vi "CTL_SpecCheckRev3.vi"(6 "Max Index":i32=12, 7 "Drain!Fill":bool, 8 "Level IN inches":dbl=5.0, 9 "Index":i32=3, 10 "ChA/!ChB":bool, 11 "Full Cfg":T3) -> (0 "Measure":dbl, 1 "Set Point":dbl, 3 "In Range?":bool=TRUE)   [LabVIEW 2024]
uses:
  Control Definitions/Ded LUT_Status.ctl
  Control Definitions/Def Spec RNG.ctl
  Control Definitions/Def Bench Status.ctl
  Control Definitions/Def PumpCtlRefs.ctl
  Control Definitions/Def BenchCfg.ctl
  Control Definitions/Def FullCfg.ctl
  Control Definitions/Def_PumpSpeed.ctl
panel:
  out "Spec Range Out":T1
  out "error out":errorcluster
  in  "error in (no error)":errorcluster
  # "In Range = TRUE when"
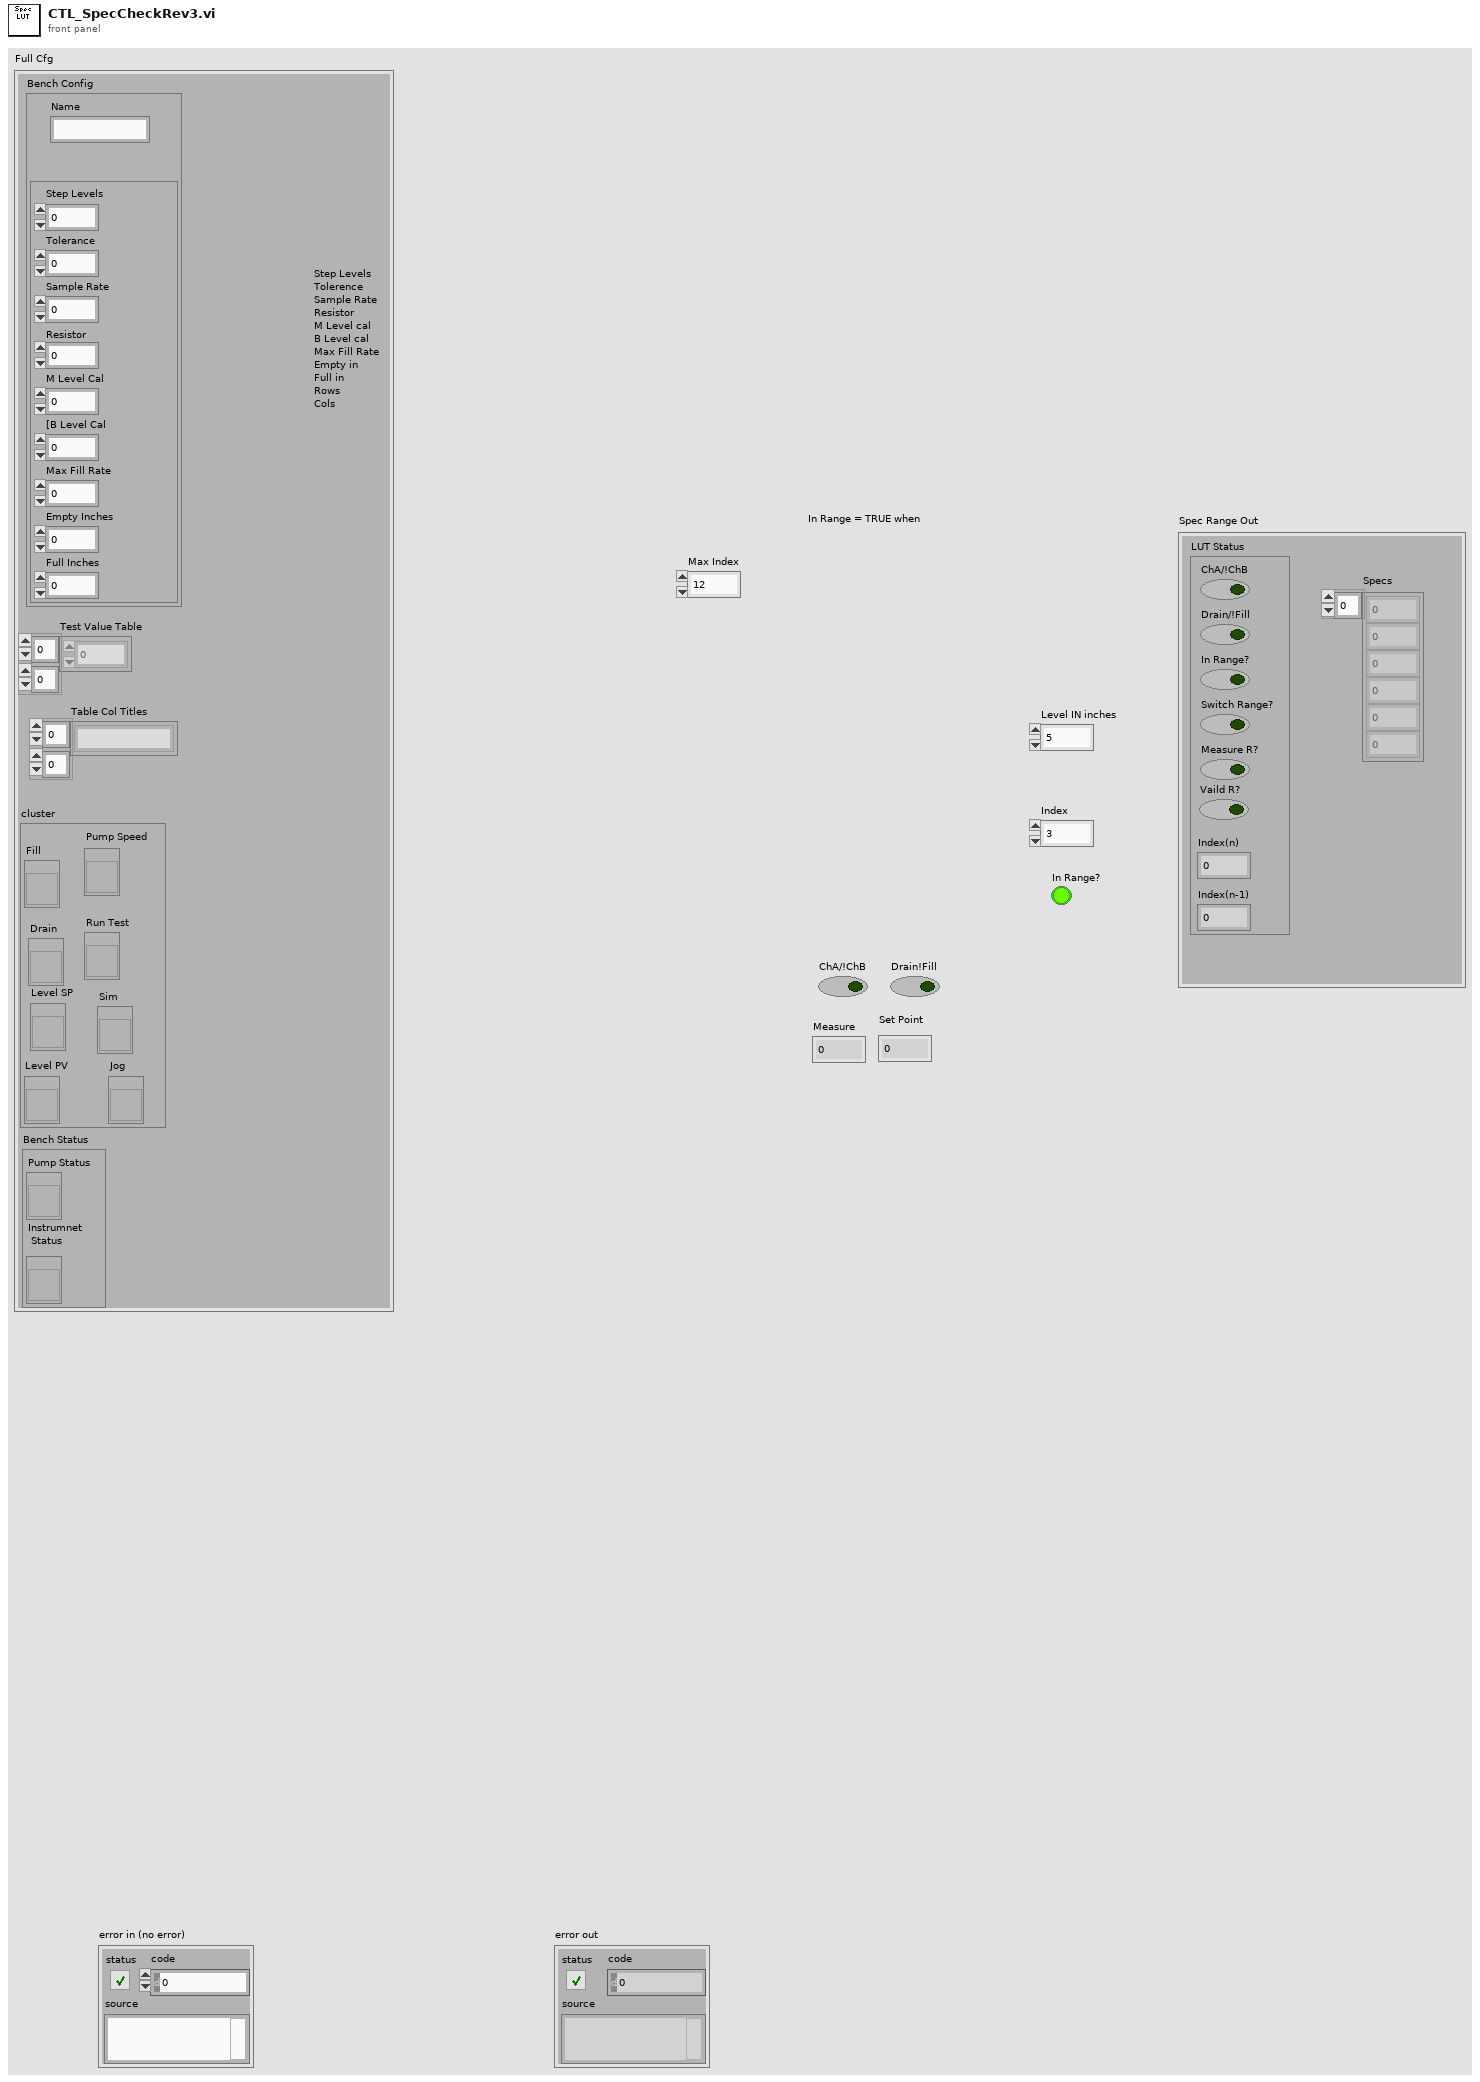
[diagram p1: front panel]
types:
  T1 = typedef "Def Spec RNG.ctl" = cluster{"Specs":dbl[], "LUT Status":T2}
  T2 = typedef "Ded LUT_Status.ctl" = cluster{"ChA/!ChB":bool, "Drain/!Fill":bool, "In Range?":bool, "Switch Range?":bool, "Measure R?":bool, "Vaild R?":bool, "Index(n)":i32, "Index(n-1)":i32}
  T3 = typedef "Def FullCfg.ctl" = cluster{"Bench Config":T4, "Test Value Table ":dbl[][], "Table Col Titles":string[][], "cluster":T5, "Bench Status":T6}
  T4 = typedef "Def BenchCfg.ctl" = cluster{"Name":string, cluster{"Step Levels":dbl, "Tolerance":dbl, "Sample Rate":dbl, "Resistor":dbl, "M Level Cal":dbl, "[B Level Cal":dbl, "Max Fill Rate":dbl, "Empty Inches":dbl, "Full Inches":dbl}}
  T5 = typedef "Def PumpCtlRefs.ctl" = cluster{"Fill ":refnum<vi>, "Drain":refnum<vi>, "Level PV":refnum<vi>, "Pump Speed":refnum<vi>, "Run Test":refnum<vi>, "Sim":refnum<vi>, "Jog":refnum<vi>, "Level SP":refnum<vi>}
  T6 = typedef "Def Bench Status.ctl" = cluster{"Pump Status":refnum<vi>, "Instrumnet\n Status":refnum<vi>}
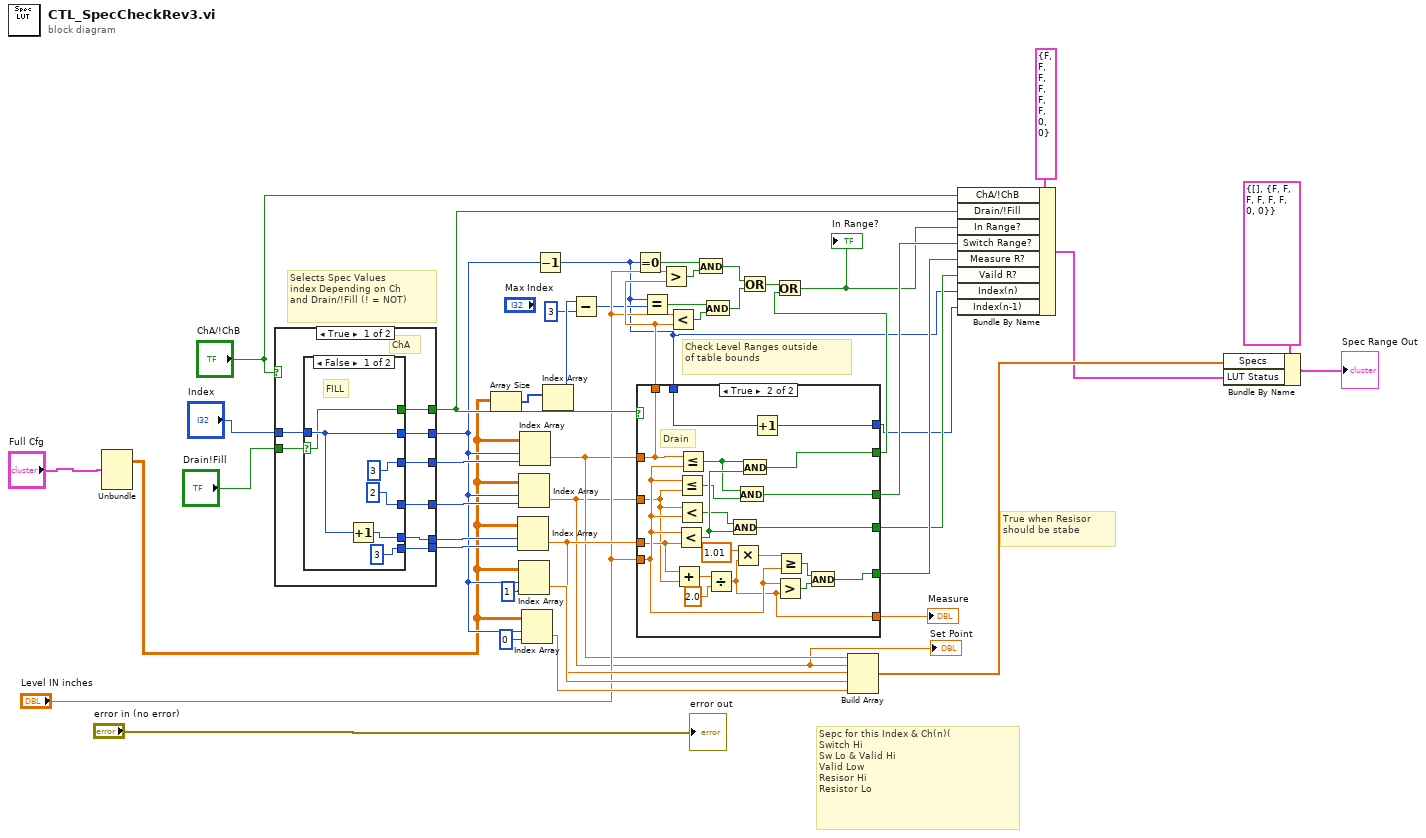
[diagram p0: block diagram]
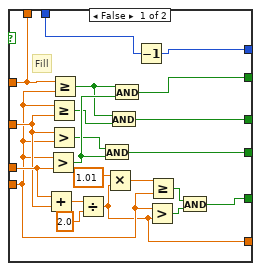
[diagram p2: hidden frame]
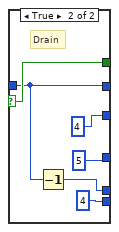
[diagram p3: hidden frame]
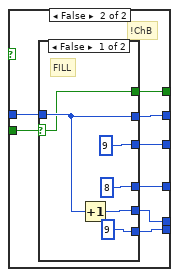
[diagram p4: hidden frame]
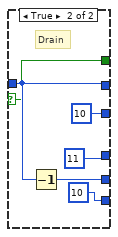
[diagram p5: hidden frame]
diagram:
  # "Selects Spec Values\nindex Depending on Ch\nand Drain/!Fill (! = NOT)"
  # "True when Resisor \nshould be stabe"
  # "Sepc for this Index & Ch(n)(\nSwitch Hi\nSw Lo & Valid Hi  \nValid Low\nResisor Hi\nResistor Lo"
  # "Check Level Ranges outside \nof table bounds"
  n1 = Unbundle("Full Cfg") -> ("Test Value Table"=w15:dbl[][])  [unwired: 4 out]
  n2 = case shown="True" "ChA/!ChB" {
    tunnel: "Drain!Fill" -> [w53 w67]
    tunnel: "Index" -> [w52 w73]
    tunnel: [w51 w72] -> w21
    tunnel: [w50 w71] -> w42
    tunnel: [w49 w70] -> w41
    tunnel: [w48 w69] -> w40
    tunnel: [w47 w68] -> w23
    tunnel: [w46 w66] -> w27
    frame True {
      # "ChA"
      n3 = case shown="False" w53 {
        selector: w53 -> [w54 w62]
        tunnel: [3 ("disabled index (col)") 4 ("disabled index (col)")] -> w47
        tunnel: [3 ("disabled index (col)") 4 ("disabled index (col)")] -> w49
        tunnel: w52 -> [w55 w60]
        tunnel: [w55 w60] -> w51
        tunnel: [w57 w61] -> w50
        tunnel: [2 ("disabled index (col)") 5 ("disabled index (col)")] -> w48
        tunnel: [w54 w62] -> w46
        frame False {
          # "FILL"
          n4 = Increment(x=w55) -> (x+1=w57:i32)
        }
        frame True {
          # "Drain"
          n5 = Decrement(x=w60) -> (x-1=w61:i32)
        }
      }
    }
    frame False {
      # "!ChB"
      n6 = case shown="False" w67 {
        selector: w67 -> [w74 w80]
        tunnel: [9 ("disabled index (col)") 10 ("disabled index (col)")] -> w68
        tunnel: [9 ("disabled index (col)") 10 ("disabled index (col)")] -> w70
        tunnel: w73 -> [w75 w81]
        tunnel: [w75 w81] -> w72
        tunnel: [w77 w83] -> w71
        tunnel: [8 ("disabled index (col)") 11 ("disabled index (col)")] -> w69
        tunnel: [w74 w80] -> w66
        frame False {
          # "FILL"
          n7 = Increment(x=w75) -> (x+1=w77:i32)
        }
        frame True {
          # "Drain"
          n8 = Decrement(x=w81) -> (x-1=w83:i32)
        }
      }
    }
  }
  n9 = Array Size(array=w15) -> (size(s)=w19:i32[])
  n10 = Index Array(array=w15, index (row)=w42, index (col)=w23) -> (element=w37:dbl)
  n11 = Index Array(array=w15, index (row)=w21, index (col)=w40) -> (element=w8:dbl)
  "Set Point" <- w8
  n12 = Index Array(array=w15, index (row)=w21, index (col)=1 ("disabled index (col)")) -> (element=w39:dbl)
  n13 = Index Array(array=w15, index (row)=w21, index (col)=w41) -> (element=w9:dbl)
  n14 = Index Array(array=w15, index (row)=w21, index (col)=0 ("disabled index (col)")) -> (element=w38:dbl)
  n15 = Decrement(x=w21) -> (x-1=w6:i32)
  n16 = Index Array(array=w19) -> (element=w18:i32)  [unwired: 1 in]
  n17 = Subtract(x=w18, y=3) -> (x-y=w16:i32)
  n18 = Equal To 0?(x=w6) -> (x = 0?=w33:bool)
  n19 = case shown="True" w27 {
    tunnel: "Level IN inches" -> [w91 w114]
    tunnel: w9 -> [w89 w112]
    tunnel: w37 -> [w99 w111]
    tunnel: [w106 w127] -> w29
    tunnel: w8 -> [w98 w110]
    tunnel: [w103 w124] -> w13
    tunnel: [w100 w121] -> w26
    tunnel: [w90 w113] -> w25
    tunnel: [w89 w112] -> w24
    tunnel: [w88 w109] -> w11
    tunnel: [w87 w108] -> w5
    tunnel: w6 -> [w86 w107]
    frame False {
      # "Fill"
      n20 = Add(x=w99, y=w98) -> (x+y=w97:dbl)
      n21 = Greater?(x=w91, y=w99) -> (0:w105:bool)
      n22 = Greater Or Equal?(x=w91, y=w98) -> (x >= y?=w101:bool)
      n23 = Greater?(x=w98, y=w91) -> (0:w104:bool)
      n24 = Greater Or Equal?(x=w89, y=w91) -> (x >= y?=w102:bool)
      n25 = Divide(x=w97, y=2.0) -> (x/y=w88:dbl)
      n26 = And(x=w104, y=w105) -> (x .and. y?=w103:bool)
      n27 = Multiply(x=1.01, y=w88) -> (x*y=w92:dbl)
      n28 = And(x=w102, y=w101) -> (x .and. y?=w100:bool)
      n29 = And(x=w102, y=w105) -> (x .and. y?=w106:bool)
      n30 = Decrement(x=w86) -> (x-1=w87:i32)
      n31 = Greater?(x=w91, y=w88) -> (0:w95:bool)
      n32 = Greater Or Equal?(x=w92, y=w91) -> (x >= y?=w94:bool)
      n33 = And(x=w94, y=w95) -> (x .and. y?=w90:bool)
    }
    frame True {
      # "Drain"
      n34 = Add(x=w111, y=w110) -> (x+y=w120:dbl)
      n35 = Less?(x=w114, y=w111) -> (x < y?=w126:bool)
      n36 = Less Or Equal?(x=w114, y=w110) -> (x <= y?=w122:bool)
      n37 = Less?(x=w110, y=w114) -> (x < y?=w125:bool)
      n38 = Less Or Equal?(x=w112, y=w114) -> (x <= y?=w123:bool)
      n39 = Divide(x=w120, y=2.0) -> (x/y=w109:dbl)
      n40 = And(x=w125, y=w126) -> (x .and. y?=w124:bool)
      n41 = Multiply(x=1.01, y=w109) -> (x*y=w115:dbl)
      n42 = And(x=w123, y=w122) -> (x .and. y?=w121:bool)
      n43 = And(x=w123, y=w126) -> (x .and. y?=w127:bool)
      n44 = Increment(x=w107) -> (x+1=w108:i32)
      n45 = Greater?(x=w114, y=w109) -> (0:w118:bool)
      n46 = Greater Or Equal?(x=w115, y=w114) -> (x >= y?=w117:bool)
      n47 = And(x=w117, y=w118) -> (x .and. y?=w113:bool)
    }
  }
  "Measure" <- w11
  n48 = Equal?(x=w6, y=w16) -> (x = y?=w35:bool)
  n49 = Greater?(x="Level IN inches", y=w24) -> (0:w34:bool)
  n50 = Less?(x="Level IN inches", y=w24) -> (x < y?=w36:bool)
  n51 = And(x=w33, y=w34) -> (x .and. y?=w31:bool)
  n52 = And(x=w35, y=w36) -> (x .and. y?=w32:bool)
  n53 = Or(x=w31, y=w32) -> (x .or. y?=w30:bool)
  n54 = Or(x=w30, y=w29) -> (x .or. y?=w14:bool)
  "In Range?" <- w14
  n55 = Build Array(w9, w8, w37, w39, w38) -> (w12:dbl[])
  n56 = Bundle By Name(cluster=T2 {"ChA/!ChB"=FALSE, "Drain/!Fill"=FALSE, "In Range?"=FALSE, "Switch Range?"=FALSE, "Measure R?"=FALSE, "Vaild R?"=FALSE, "Index(n)"=0, "Index(n-1)"=0} ("Spec Check"), "ChA/!ChB"="ChA/!ChB", "Drain/!Fill"=w27, "In Range?"=w14, "Switch Range?"=w26, "Measure R?"=w25, "Vaild R?"=w13, "Index(n)"=w6, "Index(n-1)"=w5) -> (w4:T2)
  n57 = Bundle By Name(cluster=T1 {"Specs"=[], "LUT Status"={"ChA/!ChB"=FALSE, "Drain/!Fill"=FALSE, "In Range?"=FALSE, "Switch Range?"=FALSE, "Measure R?"=FALSE, "Vaild R?"=FALSE, "Index(n)"=0, "Index(n-1)"=0}} ("Spec Range Out"), "Specs"=w12, "LUT Status"=w4) -> (→"Spec Range Out":T1)
  "error out" <- "error in (no error)"
